vi "oax_Devices Used.vi"(8 "error in":errorcluster, 11 "DAQ Config":T1 {"pregain" format="%.2f"; "IEPE" items=["On", "Off", "None"]; "coupling" items=["DC", "AC"]; "engineering units" items=["custom..."=0, "V"=1, "A"=21, "C"=30, "pC"=31, "s"=32, "-"=29, "Pa"=2, "N"=20, "g"=3, "m/s^2"=4, "m/s"=5, "m"=6, "mm/s"=12, "mm"=13, "micron/s"=14, "micron"=15, "in/s^2"=7, "in/s"=8, "in"=9, "mil/s"=10, "mil"=11, "rad/s^2"=16, "rad/s"=17, "rad"=18, "deg/s^2"=26, "deg/s"=27, "deg"=28, "RPM"=22, "cycle/s^2"=23, "Hz"=24, "cycle"=25, "strain"=19]; "sensor sensitivity (mV/EU)" format="%.2f"; "dB reference" format="%.1e"}) -> (0 "error out":errorcluster, 2 "devices used":string[](array[string]), 3 "Channels list":string)   [LabVIEW 2017]
uses:
  <vilib>/addons/Sound and Vibration/Order Analysis/Example Support/sub VIs/OAXML_DSA DAQ Config.ctl
  <vilib>/addons/_NISVFA/_Shared subVIs/Controls/svc_Engineering Units Text Ring.ctl
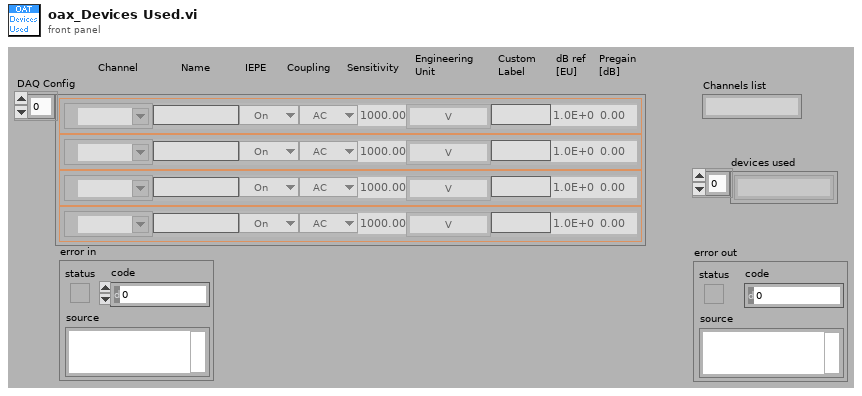
[diagram p1: front panel]
types:
  T1 = typedef "OAXML_DSA DAQ Config.ctl" = cluster{"name":string, "channel":tag, "coupling":u16, "dB reference":sgl, "sensor sensitivity (mV/EU)":dbl, "engineering units":T2, "IEPE":u16, "custom label":string, "pregain":sgl}[]
  T2 = typedef "svc_Engineering Units Text Ring.ctl" = u16
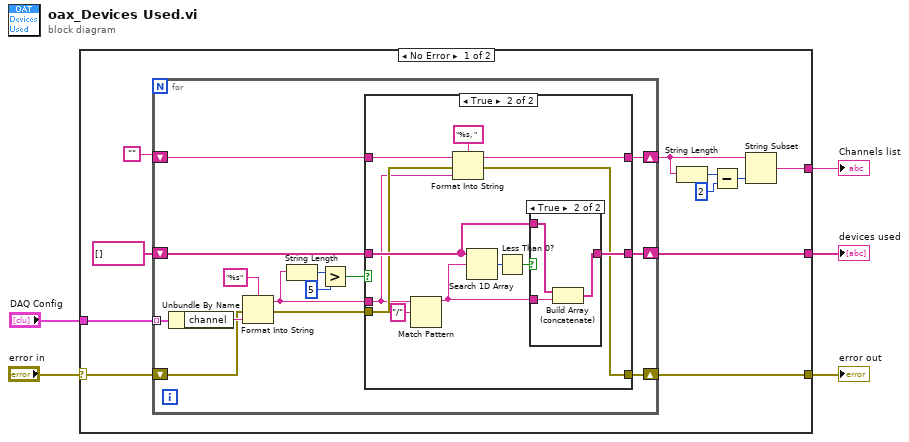
[diagram p0: block diagram]
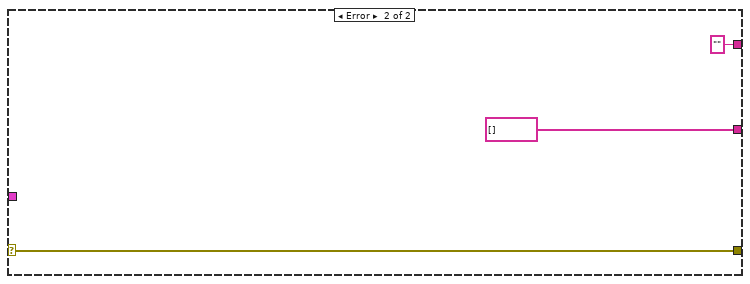
[diagram p4: hidden frame]
diagram:
  n1 = case shown="No Error" "error in" {
    selector: "error in" -> [w15 w51]
    tunnel: "DAQ Config" -> [w16 _]
    tunnel: [w13 string[] []] -> w2
    tunnel: [w12 w51] -> w3
    tunnel: [w6 ""] -> w1
    frame No Error {
      n2 = for {
        tunnel: w16 -> [w30] mode=indexing
        shift-right: [w22] -> w12
        shift-left: w15 -> [w27]
        shift-right: [w25] -> w13
        shift-left: string[] [] -> [w26]
        shift-right: [w21] -> w7
        shift-left: "" -> [w24]
        n3 = Unbundle By Name(w30) -> ("channel"=w29:tag)
        n4 = Format Into String(format string="%s", error in=w27, w29) -> (resulting string=w20:string, error out=w23:errorcluster)  [unwired: 1 in]
        n5 = String Length(string=w20) -> (length=w19:i32)
        n6 = Greater?(x=w19, y=5) -> (0:w17:bool)
        n7 = case shown="True" w17 {
          tunnel: w26 -> [w32 w43]
          tunnel: [w32 w41] -> w25
          tunnel: w24 -> [w33 w40]
          tunnel: w23 -> [w31 w37]
          tunnel: [w31 w36] -> w22
          tunnel: [w33 w35] -> w21
          tunnel: w20 -> [_ w34]
          frame False {
          }
          frame True {
            n8 = Match Pattern(string=w34, regular expression="/") -> (before substring=w39:string)  [unwired: 1 in, 3 out]
            n9 = Format Into String(format string="%s, ", initial string=w40, error in=w37, w34) -> (resulting string=w35:string, error out=w36:errorcluster)
            n10 = Search 1D Array(1D array=w43, element=w39) -> (index of element=w44:i32)  [unwired: 1 in]
            n11 = Less Than 0?(x=w44) -> (x < 0?=w42:bool)
            n12 = case shown="True" w42 {
              tunnel: w43 -> [w46 w49]
              tunnel: w39 -> [_ w48]
              tunnel: [w46 w47] -> w41
              frame False {
              }
              frame True {
                n13 = Build Array (concatenate)(w49, w48) -> (w47:string[])
              }
            }
          }
        }
      }
      n14 = String Length(string=w7) -> (length=w8:i32)
      n15 = Subtract(x=w8, y=2) -> (x-y=w9:i32)
      n16 = String Subset(string=w7, length (rest)=w9) -> (substring=w6:string)  [unwired: 1 in]
    }
    frame Error {
    }
  }
  "error out" <- w3
  "devices used" <- w2
  "Channels list" <- w1
